vi "LINX - Nonvolatile test.vi"() -> ()   [LabVIEW 2020]
uses:
  <vilib>/MakerHub/LINX/Public/Utilities/Open Serial.vi
  <vilib>/MakerHub/LINX/LMH-LINX.lvlib
panel:
  in  "stop":bool
  out "Read Device User ID 2":u16
  in  "Device User ID":u16
  in  "Set ID":bool
  in  "Serial Port":refnum<visa-resource-name>="N/A"
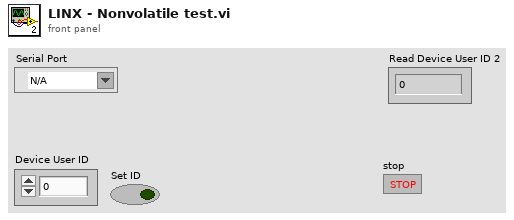
[diagram p1: front panel]
types:
  T1 = typedef "LMH-LINX.lvlib/LINX Ref.ctl" = cluster{"IO":T2, "Interface":T3, "LINX Device Config":T4}
  T2 = typedef "LMH-LINX.lvlib/Platform.ctl" = enum16{"Remote", "Local"}
  T3 = typedef "LMH-LINX.lvlib/Interface.ctl" = enum16{"Serial", "TCP"}
  T4 = typedef "LMH-LINX.lvlib/Device.lvlib/LINX Device Config.ctl" = cluster{"Interface":T3, "COM Port":refnum<visa-resource-name>, "TCP Configuration":T5, "Device Family":u8, "Device ID":u8, "Device Name":string, "TCP Ref":refnum<k5>, "Channels":T6}
  T5 = typedef "LMH-LINX.lvlib/Device.lvlib/TCP Config.ctl" = cluster{"IP Address":string, "Port":u16}
  T6 = typedef "LMH-LINX.lvlib/Channels.ctl" = cluster{"DI":u8[], "DO":u8[], "AI":u8[], "AO":u8[], "PWM":u8[], "QE":u8[], "UART":u8[], "I2C 2":u8[], "SPI":u8[], "CAN":u8[], "Servo":u8[], "AI Ref (V)":dbl, "AI Resolution (Bits)":u8, "AO Ref (V)":dbl, "AO Resolution (Bits)":u8}
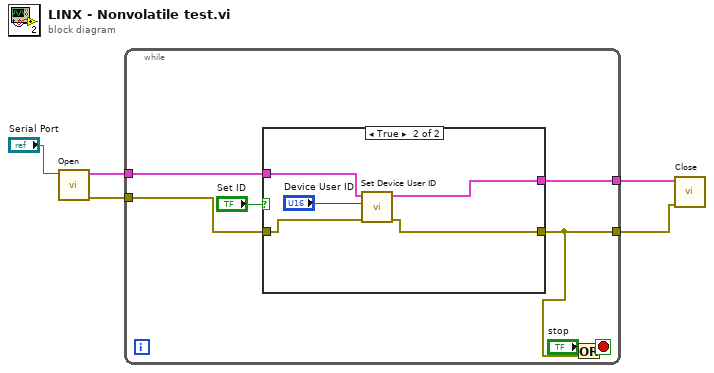
[diagram p0: block diagram]
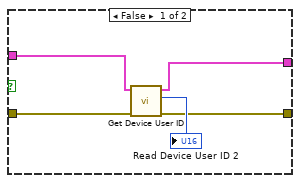
[diagram p2: hidden frame]
diagram:
  n1 = call-poly <vilib>:"Open.vi"("Serial Port"="Serial Port") -> ("Error Out"=w4:errorcluster, "LINX Resource"=w3:T1)  [unwired: 8 in, 1 out]
  n2 = while {
    tunnel: w4 -> [w11]
    tunnel: w3 -> [w10]
    tunnel: [w9] -> w2
    tunnel: [w6] -> w1
    stop <- w7 stop-if-true
    n3 = case shown="True" "Set ID" {
      tunnel: w11 -> [w16 w19]
      tunnel: w10 -> [w15 w20]
      tunnel: [w14 w21] -> w9
      tunnel: [w13 w18] -> w6
      frame False {
        n4 = call <vilib>:"Get Device User ID.vi"("Error In"=w16, "LINX Resource"=w15) -> ("Error Out"=w13:errorcluster, "Device User ID"=→"Read Device User ID 2":u16, "LINX Resource"=w14:T1)  [unwired: 7 in]
      }
      frame True {
        n5 = call <vilib>:"Set Device User ID.vi"("Error In"=w19, "Device User ID"="Device User ID", "LINX Resource"=w20) -> ("Error Out"=w18:errorcluster, "LINX Resource"=w21:T1)  [unwired: 7 in]
      }
    }
    n6 = Or(x="stop", y=w6) -> (x .or. y?=w7:bool)
  }
  n7 = call <vilib>:"Close.vi"("Error In"=w1, "LINX Resource"=w2) -> ()  [unwired: 9 in, 1 out]
